vi "Is Circle-Circle Collision.vi"(3 "Other Collider":refnum<class "Circle Collider.lvclass">, 4 "Other object in":refnum<class "SimulationObject.lvclass">, 5 "Self Collider in":refnum<class "Circle Collider.lvclass">, 6 "Self Object in":refnum<class "SimulationObject.lvclass">) -> (0 "Other Object out":refnum<class "SimulationObject.lvclass">, 1 "Are Colliding":bool, 2 "Self Object out":refnum<class "SimulationObject.lvclass">)   [LabVIEW 2022 SP3, in "Circle Collider.lvclass"]
uses:
  Circle Collider.lvclass
  SimulationObject/SimulationObject.lvclass
  SimulationObject/SimulationObject.lvclass/SimulationObject.ctl
  Components/Transform/Transform.lvclass/Transform.ctl
  Circle Collider.lvclass/Circle Collider.ctl
  Components/Transform/Transform.lvclass
  Math/Vector2/Vector2.lvclass
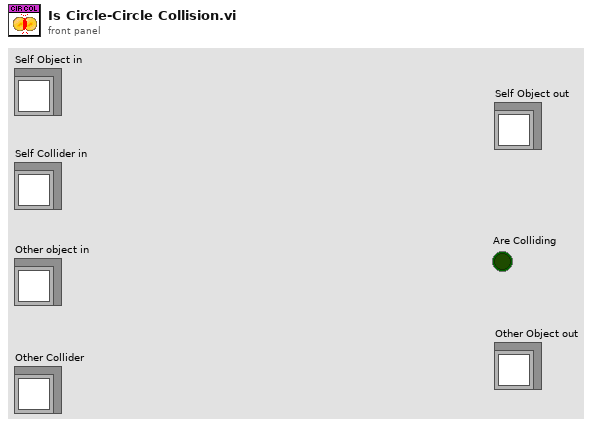
[diagram p1: front panel]
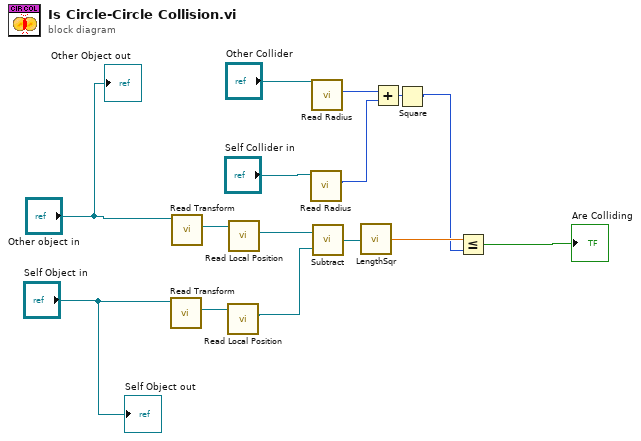
[diagram p0: block diagram]
diagram:
  n1 = call "Read Transform.vi"("SimulationObject in"="Self Object in") -> ("Transform out"=w12:refnum<class "Transform.lvclass">)  [unwired: 8 in, 2 out]
  n2 = call "Read Transform.vi"("SimulationObject in"="Other object in") -> ("Transform out"=w11:refnum<class "Transform.lvclass">)  [unwired: 8 in, 2 out]
  n3 = call "Read Local Position.vi"("Transform in"=w12) -> ("Local Position out"=w9:refnum<class "Vector2.lvclass">)  [unwired: 8 in, 2 out]
  n4 = call "Read Local Position.vi"("Transform in"=w11) -> ("Local Position out"=w10:refnum<class "Vector2.lvclass">)  [unwired: 8 in, 2 out]
  n5 = call "Read Radius.vi"("Circle Collider in"="Self Collider in") -> ("Radius"=w4:i16)  [unwired: 8 in, 2 out]
  n6 = call "Read Radius.vi"("Circle Collider in"="Other Collider") -> ("Radius"=w5:i16)  [unwired: 8 in, 2 out]
  n7 = call "Subtract.vi"("Vec2 b in"=w9, "Vec2 a in"=w10) -> ("Vec2 out"=w8:refnum<class "Vector2.lvclass">)
  n8 = call "LengthSqr.vi"("Vec2 in"=w8) -> ("Length Sqr out"=w2:sgl)
  n9 = Add(x=w5, y=w4) -> (x+y=w3:i16)
  n10 = Square(x=w3) -> (x^2=w1:i16)
  n11 = Less Or Equal?(x=w2, y=w1) -> (x <= y?=→"Are Colliding":bool)
  "Self Object out" <- "Self Object in"
  "Other Object out" <- "Other object in"
